vi "String to float array.vi"(11 "String":string) -> (3 "Array - Numeric":dbl[](array[numeric]), 5 "Array size":i32)   [LabVIEW 2020]
panel:
  in  "Array - Numeric 2":dbl[](array[numeric])
  # "Separate with comma ','\nArrays:\n1. start:stop/step\n2. start:step:stop"
  # "E.g.:\n1:6/1.8,\n4,5,6,\n1.1:0.2:3"
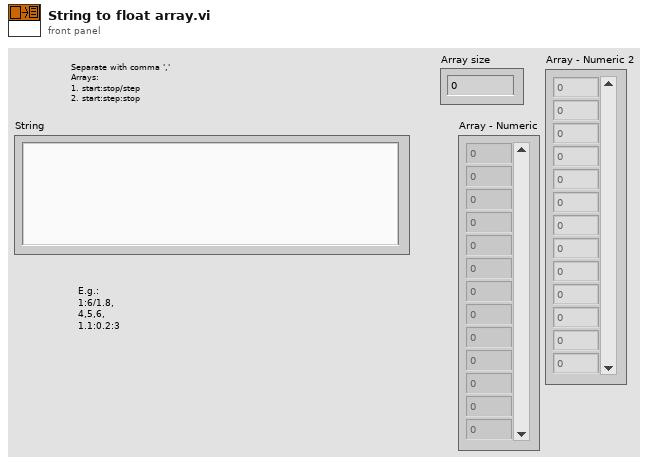
[diagram p1: front panel]
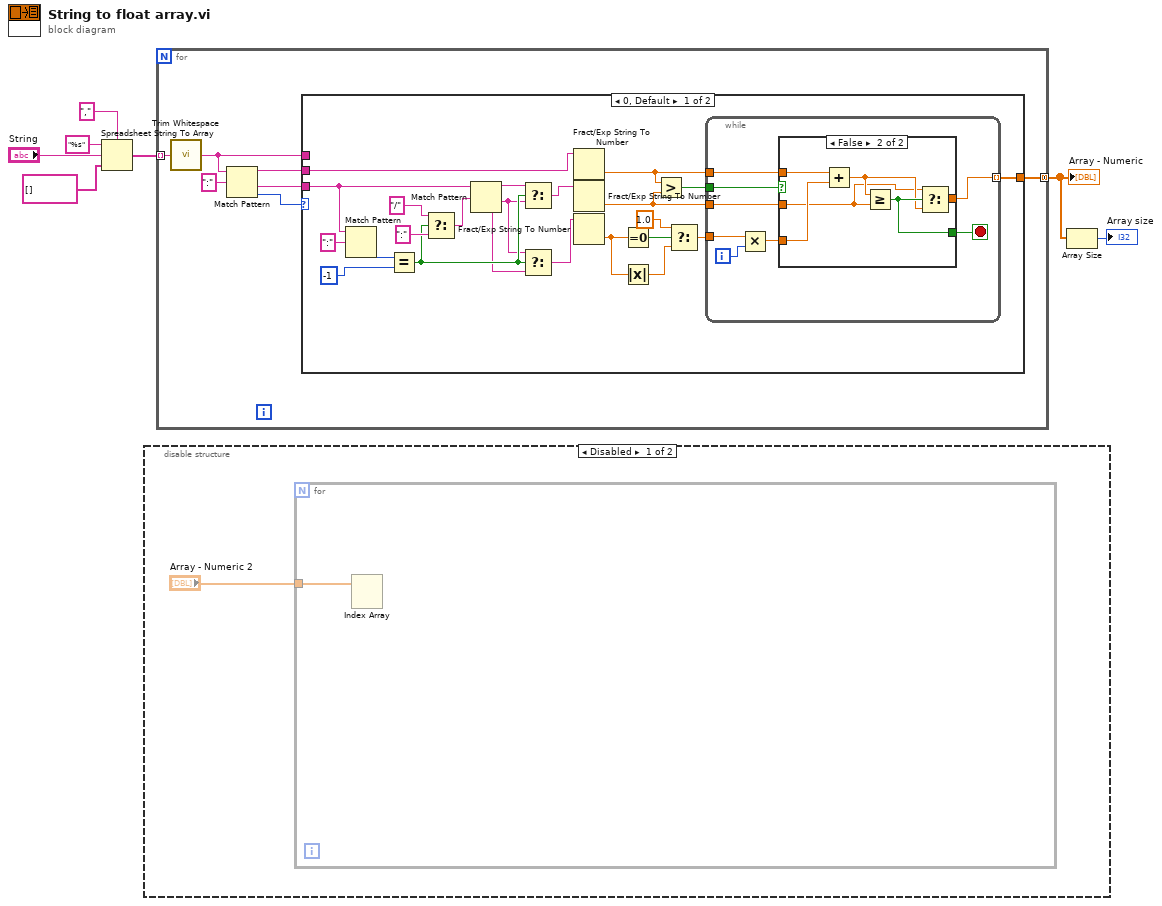
[diagram p0: block diagram]
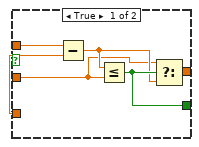
[diagram p3: hidden frame]
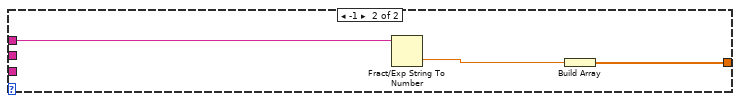
[diagram p4: hidden frame]
diagram:
  n1 = Spreadsheet String To Array(delimiter (Tab)=",", format string="%s", spreadsheet string="String", array type (2D Dbl)=string[] []) -> (array=w4:string[])
  n2 = disable-structure shown="Disabled" {
    frame Disabled {
      n3 = for {
        tunnel: "Array - Numeric 2" -> [w9]
        n4 = Index Array(array=w9) -> ()  [unwired: 2 in, 2 out]
      }
    }
    frame Enabled {
    }
  }
  n5 = for {
    tunnel: w4 -> [w12] mode=indexing
    tunnel: [w14] -> w2 mode=concatenating
    n6 = call <vilib>:"Trim Whitespace.vi"("string"=w12) -> ("trimmed string"=w11:string)  [unwired: 1 in]
    n7 = Match Pattern(string=w11, regular expression=":") -> (before substring=w13:string, after substring=w10:string, offset past match=w15:i32)  [unwired: 1 in, 1 out]
    n8 = case shown="0, Default" w15 {
      tunnel: w11 -> [_ w61]
      tunnel: [w37 w59] -> w14
      tunnel: w13 -> [w38 _]
      tunnel: w10 -> [w26 _]
      frame 0, Default {
        n9 = Match Pattern(string=w26, regular expression=":") -> (offset past match=w28:i32)  [unwired: 1 in, 3 out]
        n10 = Equal?(x=w28, y=-1) -> (x = y?=w20:bool)
        n11 = Select(t="/" ("regular expression"), s=w20, f=":") -> (s? t:f=w23:string)
        n12 = Match Pattern(string=w26, regular expression=w23) -> (before substring=w19:string, after substring=w18:string)  [unwired: 1 in, 2 out]
        n13 = Select(t=w19, s=w20, f=w18) -> (s? t:f=w21:string)
        n14 = Select(t=w18, s=w20, f=w19) -> (s? t:f=w17:string)
        n15 = Fract/Exp String To Number(string=w38) -> (number=w32:dbl)  [unwired: 3 in, 1 out]
        n16 = Fract/Exp String To Number(string=w21) -> (number=w33:dbl)  [unwired: 3 in, 1 out]
        n17 = Fract/Exp String To Number(string=w17) -> (number=w30:dbl)  [unwired: 3 in, 1 out]
        n18 = Equal To 0?(x=w30) -> (x = 0?=w36:bool)
        n19 = Absolute Value(x=w30) -> (abs(x)=w29:dbl)
        n20 = Greater?(x=w32, y=w33) -> (0:w31:bool)
        n21 = Select(t=1.0, s=w36, f=w29) -> (s? t:f=w35:dbl)
        n22 = while {
          tunnel: w32 -> [w44]
          tunnel: w35 -> [w45]
          tunnel: [w41] -> w37 mode=indexing
          tunnel: w33 -> [w40]
          tunnel: w31 -> [w39]
          i -> [w46]
          stop <- w42 stop-if-true
          n23 = Multiply(x=w45, y=w46) -> (x*y=w43:dbl)
          n24 = case shown="False" w39 {
            tunnel: w44 -> [w52 w58]
            tunnel: w43 -> [w51 w57]
            tunnel: [w50 w56] -> w42
            tunnel: [w48 w54] -> w41
            tunnel: w40 -> [w47 w53]
            frame True {
              n25 = Subtract(x=w52, y=w51) -> (x-y=w49:dbl)
              n26 = Less Or Equal?(x=w49, y=w47) -> (x <= y?=w50:bool)
              n27 = Select(t=w47, s=w50, f=w49) -> (s? t:f=w48:dbl)
            }
            frame False {
              n28 = Add(x=w58, y=w57) -> (x+y=w55:dbl)
              n29 = Greater Or Equal?(x=w55, y=w53) -> (x >= y?=w56:bool)
              n30 = Select(t=w53, s=w56, f=w55) -> (s? t:f=w54:dbl)
            }
          }
        }
      }
      frame -1 {
        n31 = Fract/Exp String To Number(string=w61) -> (number=w60:dbl)  [unwired: 3 in, 1 out]
        n32 = Build Array(w60) -> (w59:dbl[])
      }
    }
  }
  "Array - Numeric" <- w2
  n33 = Array Size(array=w2) -> (size(s)=→"Array size":i32)
